vi "VISA_QueryICannotBeStopped.vi"(9 "Numeric":i32, 11 "VISA Refnum in":refnum<visa-resource-name>) -> (0 "Chamber Pressure 2 (mbar)":dbl format="%.2f", 1 "Scroll Pump Pressure (mBar)":string, 2 "Chamber Pressure (mBar)":string, 3 "VISA Refnum out":refnum<visa-resource-name>, 8 "Scroll Pump Pressure 2 (mbar)":dbl format="%.2f")   [LabVIEW 2016]
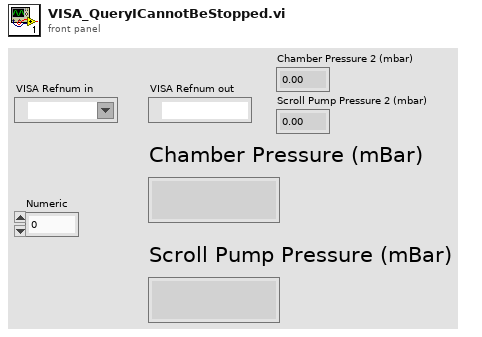
[diagram p1: front panel]
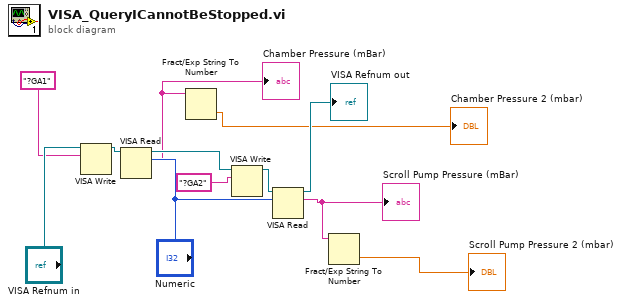
[diagram p0: block diagram]
diagram:
  n1 = VISA Write(VISA resource name="VISA Refnum in", write buffer="?GA1") -> (VISA resource name out=w8:refnum<visa-resource-name>)  [unwired: 1 in, 2 out]
  n2 = VISA Read(VISA resource name=w8, byte count="Numeric") -> (VISA resource name out=w10:refnum<visa-resource-name>, read buffer=w4:string)  [unwired: 1 in, 2 out]
  "Chamber Pressure (mBar)" <- w4
  n3 = Fract/Exp String To Number(string=w4) -> (number=→"Chamber Pressure 2 (mbar)":dbl)  [unwired: 3 in, 1 out]
  n4 = VISA Write(VISA resource name=w10, write buffer="?GA2") -> (VISA resource name out=w9:refnum<visa-resource-name>)  [unwired: 1 in, 2 out]
  n5 = VISA Read(VISA resource name=w9, byte count="Numeric") -> (VISA resource name out=→"VISA Refnum out":refnum<visa-resource-name>, read buffer=w2:string)  [unwired: 1 in, 2 out]
  "Scroll Pump Pressure (mBar)" <- w2
  n6 = Fract/Exp String To Number(string=w2) -> (number=→"Scroll Pump Pressure 2 (mbar)":dbl)  [unwired: 3 in, 1 out]
